vi "JSON to Dependency.vi"(11 "Dependency JSON":string) -> (3 "Dependency":T1)   [LabVIEW 2020, in "neg-pkg.lvlib" / "Package.lvclass"]
uses:
  Package.lvclass
  Dependency.ctl
  Package ID.ctl
  Package Type.ctl
  neg_pkgs/negentropicdev/lv-json/JSON/JSON.lvlib
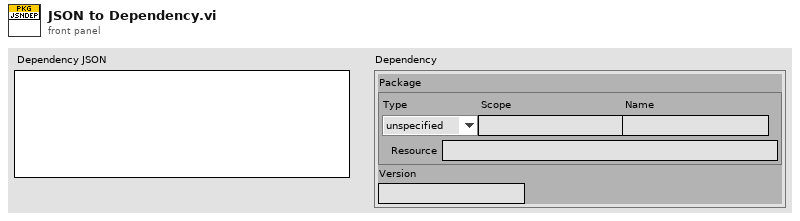
[diagram p1: front panel]
types:
  T1 = typedef "neg-pkg.lvlib/Package.lvclass/Dependency.ctl" = cluster{"Package":T2, "Version":string}
  T2 = typedef "neg-pkg.lvlib/Package.lvclass/Package ID.ctl" = cluster{"Type":T3, "Scope":string, "Name":string, "Resource":string}
  T3 = typedef "neg-pkg.lvlib/Package.lvclass/Package Type.ctl" = enum16{"unspecified", "git"}
  T4 = typedef "JSON.lvlib/JSON Item Type.ctl" = enum16{"unknown", "null", "Array", "Object", "String", "Number", "Boolean"}
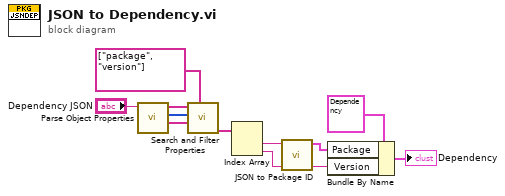
[diagram p0: block diagram]
diagram:
  n1 = call "Parse Object Properties.vi"("JSON String"="Dependency JSON") -> ("Values"=w8:string[], "Item Types"=w9:T4[], "Keys"=w10:string[])  [unwired: 7 in, 1 out]
  n2 = call "Search and Filter Properties.vi"("Search Keys"=string[] ["package", "version"], "Values In"=w8, "Types In"=w9, "Keys In"=w10) -> ("Filtered Values"=w6:string[])  [unwired: 2 in, 5 out]
  n3 = Index Array(array=w6) -> (element #1=w5:string, element #2=w1:string)  [unwired: 2 in]
  n4 = call "JSON to Package ID.vi"("JSON"=w5) -> ("Package"=w2:T2)  [unwired: 10 in]
  n5 = Bundle By Name(cluster=T1 {"Package"={"Type"=enum."git", "Scope"="negentropicdev", "Name"="lv-json", "Resource"=""}, "Version"=""} ("Dependency"), "Package"=w2, "Version"=w1) -> (→"Dependency":T1)
